vi "events test.vi"   [LabVIEW 2015]
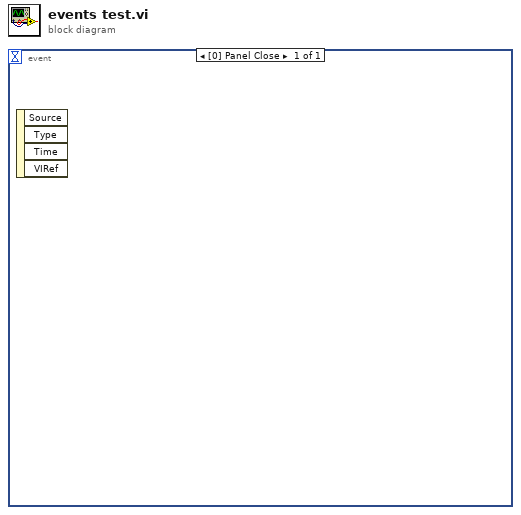
[diagram p0: block diagram]
diagram:
  n1 = event shown="[0] Panel Close" {
    selector: _ -> [_]
    dyn-events: _ -> [_]
    timeout: _ -> [_]
    event Panel Close {
      n2 = event-data() -> ()  [unwired: 1 in, 4 out]
    }
  }
